vi "ATS_String_To_Value.vi"(7 "String_In":string) -> (2 "Value_Out":dbl format="%.2f", 3 "Text_Out":string)   [LabVIEW 2014]
doc: "_____AlazarTech, Scope_____\n\nConvert the CLock Rate control to Numerical and Text value."
panel:
  in  "In_Value":dbl format="%.2p"
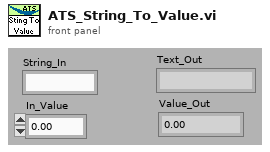
[diagram p1: front panel]
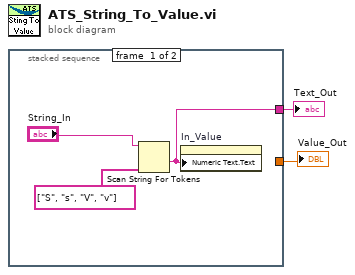
[diagram p0: block diagram]
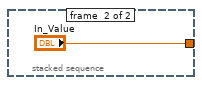
[diagram p2: hidden frame]
diagram:
  n1 = stacked-sequence {
    tunnel: [w4 _] -> w2
    tunnel: [_ "In_Value"] -> w1
    frame #0 {
      n2 = Scan String For Tokens(6:string[] ["S", "s", "V", "v"] ("delimiters (\\s,\\t,\\r,\\n)"), 9:"String_In") -> (1:w4:string)  [unwired: 4 in, 3 out]
      n3 = property on="In_Value" class="DigNum (strict)"("Numeric Text.Text"=w4) -> ()  [unwired: 2 in, 2 out]
    }
    frame #1 {
    }
  }
  "Text_Out" <- w2
  "Value_Out" <- w1
